vi "ATF-Pump-TC waveform Samples bulider.vi"(7 "Samples":i32=10, 9 "Data input":waveform(dbl)[](array[waveform]), 11 "RD.TC_Data RD":refnum<queue>) -> (1 "Data out":waveform(dbl)[](array[waveform]))   [LabVIEW 2022 SP3]
panel:
  out "overflow?":bool
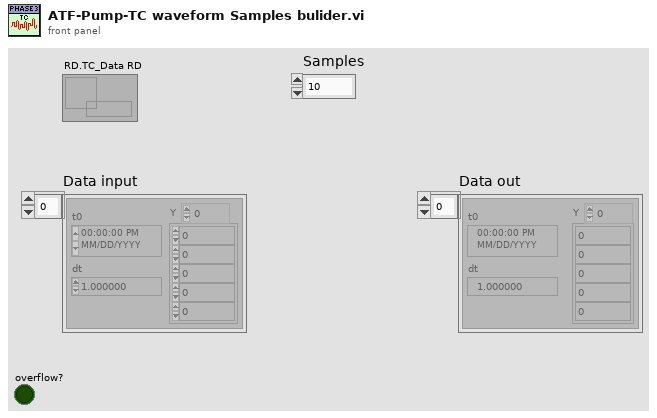
[diagram p1: front panel]
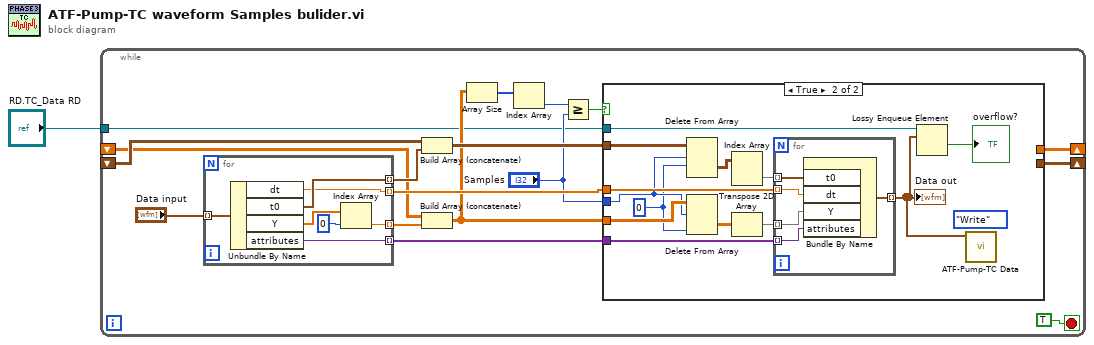
[diagram p0: block diagram]
diagram:
  n1 = while {
    shift-right: [w5] -> _
    shift-left: _ -> [w6]
    shift-right: [w3] -> _
    shift-left: _ -> [w4]
    tunnel: "RD.TC_Data RD" -> [w2]
    stop <- TRUE stop-if-true
    n2 = for {
      tunnel: "Data input" -> [w45] mode=indexing
      tunnel: [w43] -> w9 mode=indexing
      tunnel: [w41] -> w15 mode=indexing
      tunnel: [w40] -> w17 mode=indexing
      tunnel: [w39] -> w18 mode=indexing
      n3 = Unbundle By Name(w45) -> ("dt"=w39:dbl, "t0"=w41:timestamp, "Y"=w44:dbl[], "attributes"=w40:variant)
      n4 = Index Array(array=w44, index=0) -> (element=w43:dbl)
    }
    n5 = Build Array (concatenate)(w6, w15) -> (w16:timestamp[][])
    n6 = Build Array (concatenate)(w4, w9) -> (w12:dbl[][])
    n7 = Array Size(array=w12) -> (size(s)=w10:i32[])
    n8 = Index Array(array=w10) -> (element=w11:i32)  [unwired: 1 in]
    n9 = Greater Or Equal?(x=w11, y="Samples") -> (x >= y?=w13:bool)
    n10 = case shown="True" w13 {
      tunnel: w12 -> [w20 w33]
      tunnel: [w20 _] -> w3
      tunnel: w16 -> [w19 w31]
      tunnel: [w19 _] -> w5
      tunnel: w17 -> [_ w28]
      tunnel: w18 -> [_ w26]
      tunnel: "Samples" -> [_ w25]
      tunnel: w2 -> [_ w23]
      frame False {
      }
      frame True {
        (unwired) enum16{"Write", "Read"}."Write" ("Enum")
        w24 = 0 ("index (row)")
        n11 = Delete From Array(array=w31, length=w25, index (row)=w24) -> (deleted portion=w30:timestamp[][])  [unwired: 1 in, 1 out]
        n12 = Delete From Array(array=w33, length=w25, index (col)=w24) -> (deleted portion=w32:dbl[][])  [unwired: 1 in, 1 out]
        n13 = Index Array(array=w30) -> (element=w29:timestamp[])  [unwired: 2 in]
        n14 = Transpose 2D Array(2D array=w32) -> (transposed array=w27:dbl[][])
        n15 = for {
          tunnel: w27 -> [w38] mode=indexing
          tunnel: w29 -> [w37] mode=indexing
          tunnel: w28 -> [w36] mode=indexing
          tunnel: [w35] -> w21 mode=indexing
          tunnel: w26 -> [w34] mode=indexing
          n16 = Bundle By Name("t0"=w37, "dt"=w34, "Y"=w38, "attributes"=w36) -> (w35:waveform(dbl))  [unwired: 1 in]
        }
        "Data out" <- w21
        n17 = Lossy Enqueue Element(queue=w23, element=w21) -> (overflow?=→"overflow?":bool)  [unwired: 1 in, 3 out]
        n18 = call "ATF-Pump-TC Data.vi"("In_TC data"=w21) -> ()  [unwired: 10 in, 1 out]
      }
    }
  }
